vi "Create Coverage Report - Lines are Hit when Covered.vi"() -> ()   [LabVIEW 2017, in "Cobertura.Tests.lvlib"]
uses:
  Cobertura.Tests.lvlib
  Cobertura/Coverage/Coverage.lvclass/Coverage.ctl
  Cobertura/Package/Package.lvclass/Package.ctl
  Cobertura/Class/Class.lvclass/Class.ctl
  Cobertura/Method/Method.lvclass/Method.ctl
  Cobertura/Line/Line.lvclass/Line.ctl
  Cobertura/Line/Read Hits.vi
  Cobertura/Coverage/Read Packages.vi
  Cobertura/Package/Read Classes.vi
  Cobertura/Class/Read Methods.vi
  Cobertura/Method/Read Lines.vi
  Fake Project Inspector/Fake Project Inspector.lvclass
  C:/Users/Pascal/Projects/Home/lvunit/Cobertura/Project Inspector Base/Project Inspector Base.lvclass
  Fake Code Coverage/Fake Code Coverage.lvclass
  C:/Users/Pascal/Projects/Home/lvunit/Code Coverage/Code Coverage.lvclass
  Fake Code Inspector/Fake Code Inspector.lvclass
  C:/Users/Pascal/Projects/Home/lvunit/Cobertura/Code Inspector Base/Code Inspector Base.lvclass
  Cobertura/Package/Package.lvclass
  Cobertura/Class/Class.lvclass
  Cobertura/Method/Method.lvclass
  Cobertura/Line/Line.lvclass
  Cobertura/Cobertura.lvlib
  <vilib>/PNR/Transparent Assertions/Transparent Assertions/Transparent Assertions.lvlib
  Cobertura/Coverage/Coverage.lvclass
panel:
  out "error out":errorcluster
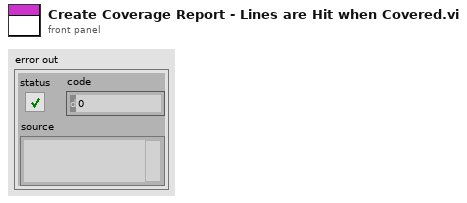
[diagram p1: front panel]
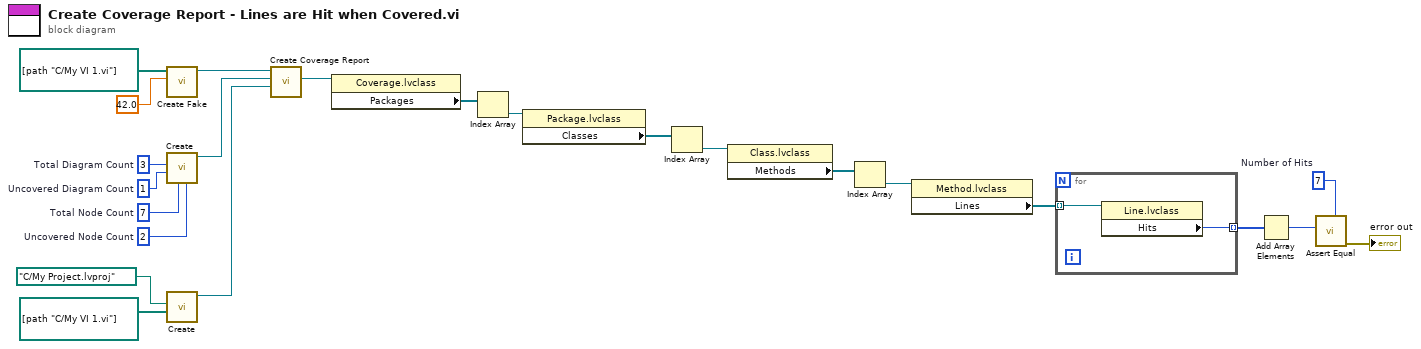
[diagram p0: block diagram]
diagram:
  w4 = 2  # Uncovered Node Count
  w5 = 7  # Total Node Count
  w6 = 1  # Uncovered Diagram Count
  w7 = 3  # Total Diagram Count
  w11 = u32 7  # Number of Hits
  n1 = call "Create Fake.vi"("Coverage Percentage"=42.0, "All VIs Measured"=path[] [path "C:/My VI 1.vi"] ("Item Paths")) -> ("Fake Code Coverage"=w13:refnum<class "Fake Code Coverage.lvclass">)  [unwired: 8 in, 1 out]
  n2 = call "Create.vi"("Uncovered Node Count"=w4, "Total Node Count"=w5, "Uncovered Diagram Count"=w6, "Total Diagram Count"=w7) -> ("Fake Code Inspector"=w8:refnum<class "Fake Code Inspector.lvclass">)  [unwired: 6 in, 1 out]
  n3 = call "Create.vi"("Item Paths"=path[] [path "C:/My VI 1.vi"], "Path"=path "C:/My Project.lvproj") -> ("Fake Project Inspector"=w21:refnum<class "Fake Project Inspector.lvclass">)  [unwired: 8 in, 1 out]
  n4 = call "Create Coverage Report.vi"("Project Inspector"=w21, "Code Inspector"=w8, "CodeCoverage in"=w13) -> ("Coverage"=w23:refnum<class "Coverage.lvclass">)  [unwired: 7 in, 1 out]
  n5 = property class="Coverage.lvclass"(reference=w23) -> ("Packages"=w22:refnum<class "Package.lvclass">[])  [unwired: 1 in, 2 out]
  n6 = Index Array(array=w22) -> (element=w19:refnum<class "Package.lvclass">)  [unwired: 1 in]
  n7 = property class="Package.lvclass"(reference=w19) -> ("Classes"=w18:refnum<class "Class.lvclass">[])  [unwired: 1 in, 2 out]
  n8 = Index Array(array=w18) -> (element=w16:refnum<class "Class.lvclass">)  [unwired: 1 in]
  n9 = property class="Class.lvclass"(reference=w16) -> ("Methods"=w15:refnum<class "Method.lvclass">[])  [unwired: 1 in, 2 out]
  n10 = Index Array(array=w15) -> (element=w14:refnum<class "Method.lvclass">)  [unwired: 1 in]
  n11 = property class="Method.lvclass"(reference=w14) -> ("Lines"=w3:refnum<class "Line.lvclass">[])  [unwired: 1 in, 2 out]
  n12 = for {
    tunnel: [w25] -> w9 mode=indexing
    tunnel: w3 -> [w24] mode=indexing
    n13 = property class="Line.lvclass"(reference=w24) -> ("Hits"=w25:u32)  [unwired: 1 in, 2 out]
  }
  n14 = Add Array Elements(numeric array=w9) -> (sum=w2:u32)
  n15 = call <vilib>:"Assert Equal.vi"("Expected"=w11, "Actual"=w2) -> ("error out"=→"error out":errorcluster)  [unwired: 9 in]
